vi "UMLEditor_ReadXmiFile_AnalyseAssText.vi"(1 "text":string="\t<memberEnd xmi:idref=\"EAID_dstB66838_A6D7_4f82_9283_F2214000E925\"/>\n\t\t\t\t\t<ownedEnd xmi:type=\"uml:Property\" xmi:id=\"EAID_dstB66838_A6D7_4f82_9283_F2214000E925\" visibility=\"public\" association=\"EAID_F3B66838_A6D7_4f82_9283_F2214000E925\" isStatic=\"false\" isReadOnly=\"false\" isDerived=\"false\" isOrdered=\"false\" isUnique=\"true\" isDerivedUnion=\"false\" aggregation=\"none\">\n\t\t\t\t\t\t<type xmi:idref=\"EAID_BDBB4C97_A1E7_4ecc_B5E2_52D4EA971126\"/>\n\t\t\t\t\t</ownedEnd>\n\t\t\t\t\t<memberEnd xmi:idref=\"EAID_srcB66838_A6D7_4f82_9283_F2214000E925\"/>\n\t\t\t\t\t<ownedEnd xmi:type=\"uml:Property\" xmi:id=\"EAID_srcB66838_A6D7_4f82_9283_F2214000E925\" visibility=\"public\" association=\"EAID_F3B66838_A6D7_4f82_9283_F2214000E925\" isStatic=\"false\" isReadOnly=\"false\" isDerived=\"false\" isOrdered=\"false\" isUnique=\"true\" isDerivedUnion=\"false\" aggregation=\"none\">\n\t\t\t\t\t\t<type xmi:idref=\"EAID_08B756DE_5C06_4edc_9F0A_D17F3D5FFCDA\"/>\n\t\t\t\t\t</ownedEnd>") -> (0 "Association":T1)   [LabVIEW 2020]
uses:
  <resource>/Framework/Providers/Open_GDS/UML/UMLEditor/UMLEditor_ReadXmiFile_Association.ctl
  <resource>/Framework/Providers/Open_GDS/UML/UMLEditor/UMLEditor_ReadXmiFile_AssType.ctl
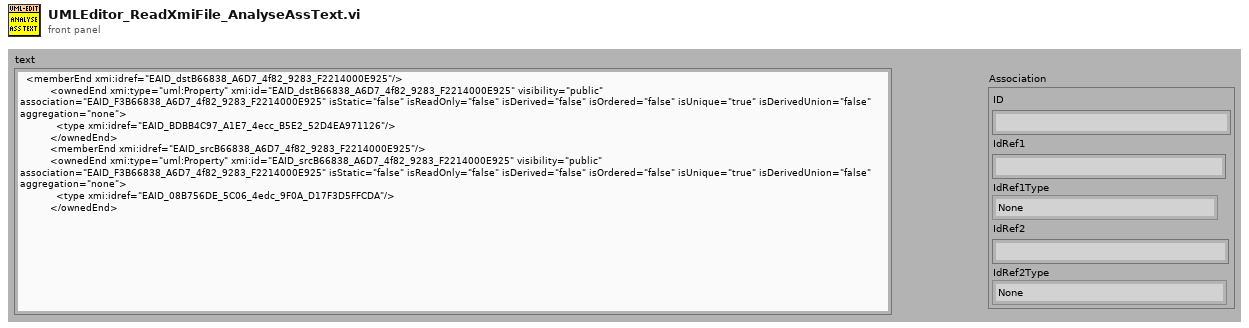
[diagram p1: front panel]
types:
  T1 = typedef "UMLEditor_ReadXmiFile_Association.ctl" = cluster{"ID":string, "IdRef1":string, "IdRef1Type":T2, "IdRef2":string, "IdRef2Type":T2}
  T2 = typedef "UMLEditor_ReadXmiFile_AssType.ctl" = enum16{"None", "Shared", "Composite"}
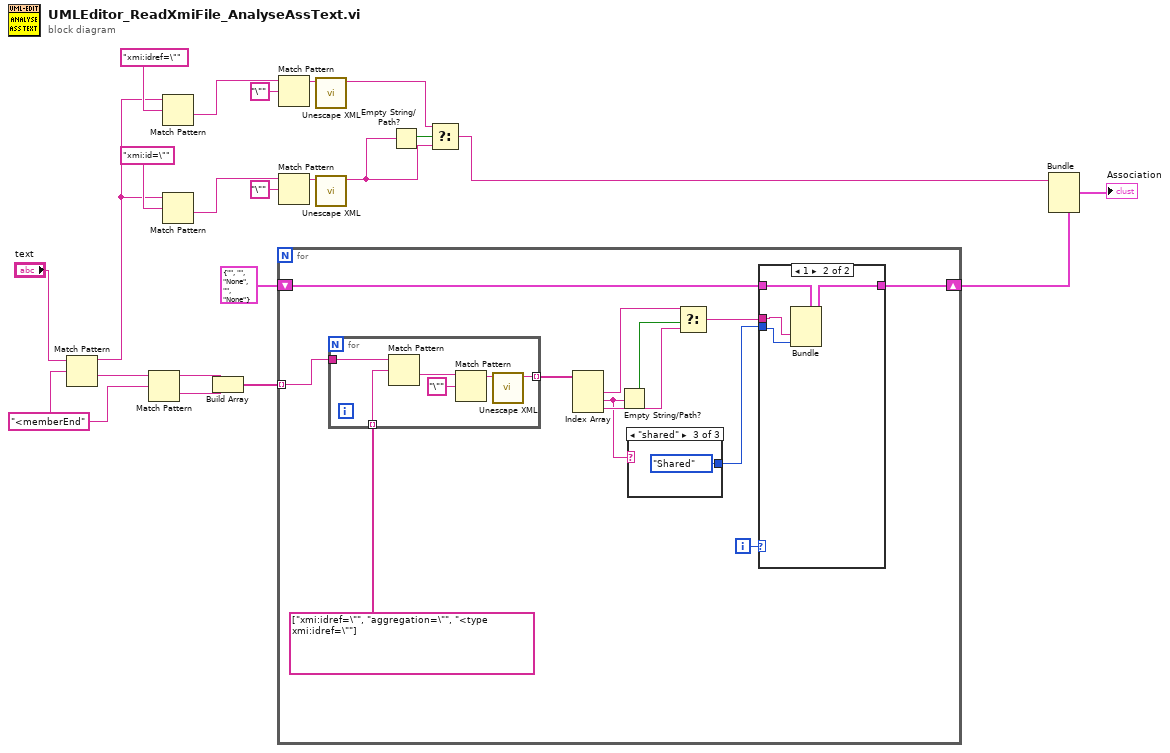
[diagram p0: block diagram]
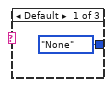
[diagram p2: hidden frame]
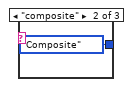
[diagram p3: hidden frame]
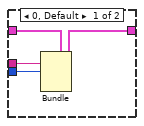
[diagram p4: hidden frame]
diagram:
  w20 = "<memberEnd"
  n1 = Match Pattern(string="text", regular expression=w20) -> (before substring=w5:string, after substring=w21:string)  [unwired: 1 in, 2 out]
  n2 = Match Pattern(string=w21, regular expression=w20) -> (before substring=w19:string, after substring=w18:string)  [unwired: 1 in, 2 out]
  n3 = Match Pattern(string=w5, regular expression="xmi:idref=\"") -> (after substring=w9:string)  [unwired: 1 in, 3 out]
  n4 = Match Pattern(string=w5, regular expression="xmi:id=\"") -> (after substring=w12:string)  [unwired: 1 in, 3 out]
  n5 = Build Array(w19, w18) -> (w17:string[])
  n6 = for {
    tunnel: w17 -> [w32] mode=indexing
    shift-right: [w23] -> w10
    shift-left: T1 {"ID"="", "IdRef1"="", "IdRef1Type"=enum."None", "IdRef2"="", "IdRef2Type"=enum."None"} ("Association") -> [w30]
    i -> [w31]
    n7 = for {
      tunnel: string[] ["xmi:idref=\"", "aggregation=\"", "<type xmi:idref=\""] -> [w51] mode=indexing
      tunnel: w32 -> [w50]
      tunnel: [w46] -> w33 mode=indexing
      n8 = Match Pattern(string=w50, regular expression=w51) -> (after substring=w49:string)  [unwired: 1 in, 3 out]
      n9 = Match Pattern(string=w49, regular expression="\"") -> (before substring=w47:string)  [unwired: 1 in, 3 out]
      n10 = call <vilib>:"Unescape XML.vi"("XML String In"=w47) -> ("XML String Out"=w46:string)  [unwired: 9 in, 1 out]
    }
    n11 = Index Array(array=w33) -> (element #1=w29:string, element #2=w25:string, element #3=w27:string)  [unwired: 3 in]
    n12 = Empty String/Path?(string/path=w25) -> (empty?=w26:bool)
    n13 = case shown="\"shared\"" w25 {
      tunnel: [UMLEditor_ReadXmiFile_AssType."None" ("IdRef2Type") UMLEditor_ReadXmiFile_AssType."Composite" ("IdRef2Type") UMLEditor_ReadXmiFile_AssType."Shared" ("IdRef2Type")] -> w24
      frame Default {
      }
      frame "composite" {
      }
      frame "shared" {
      }
    }
    n14 = Select(t=w29, s=w26, f=w27) -> (s? t:f=w28:string)
    n15 = case shown="1" w31 {
      tunnel: w28 -> [w40 w43]
      tunnel: w30 -> [w41 w45]
      tunnel: w24 -> [w39 w42]
      tunnel: [w38 w44] -> w23
      frame 0, Default {
        n16 = Bundle(cluster=w41, "IdRef1"=w40, "IdRef1Type"=w39) -> (w38:T1)  [unwired: 3 in]
      }
      frame 1 {
        n17 = Bundle(cluster=w45, "IdRef2"=w43, "IdRef2Type"=w42) -> (w44:T1)  [unwired: 3 in]
      }
    }
  }
  n18 = Match Pattern(string=w9, regular expression="\"") -> (before substring=w7:string)  [unwired: 1 in, 3 out]
  n19 = Match Pattern(string=w12, regular expression="\"") -> (before substring=w14:string)  [unwired: 1 in, 3 out]
  n20 = call <vilib>:"Unescape XML.vi"("XML String In"=w7) -> ("XML String Out"=w3:string)  [unwired: 9 in, 1 out]
  n21 = call <vilib>:"Unescape XML.vi"("XML String In"=w14) -> ("XML String Out"=w2:string)  [unwired: 9 in, 1 out]
  n22 = Empty String/Path?(string/path=w2) -> (empty?=w4:bool)
  n23 = Select(t=w3, s=w4, f=w2) -> (s? t:f=w1:string)
  n24 = Bundle(cluster=w10, "ID"=w1) -> (→"Association":T1)  [unwired: 4 in]
